vi "rad_Check Firmware.vi"(8 "error in (no error)":errorcluster, 11 "System Configuration":refnum<k21>) -> (0 "error out":errorcluster, 3 "System Configuration out":refnum<k21>, 4 "Bad firmware and user canceled":bool)   [LabVIEW 2016]
uses:
  <resource>/objmgr/nisysapi.rc
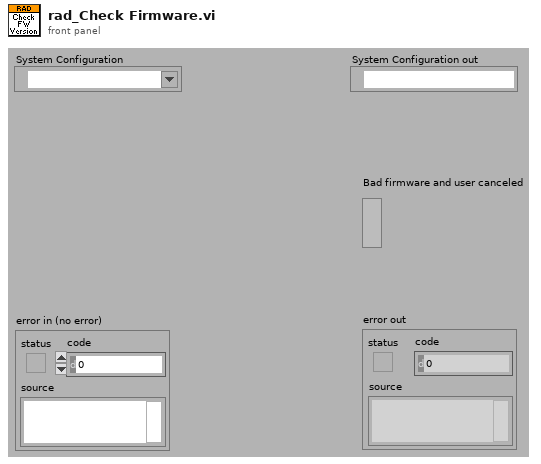
[diagram p1: front panel]
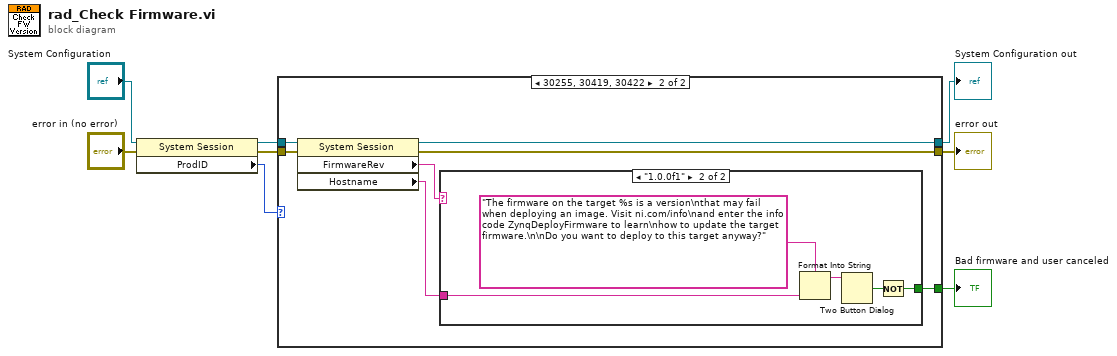
[diagram p0: block diagram]
diagram:
  n1 = property class="System Session"(reference="System Configuration", error in="error in (no error)") -> (reference out=w4:refnum<k21>, error out=w3:errorcluster, "ProdID"=w6:i32)
  n2 = case shown="30255, 30419, 30422" w6 {
    tunnel: [_ w17] -> w5
    tunnel: w4 -> [w10 w16]
    tunnel: w3 -> [w9 w15]
    tunnel: [w10 w14] -> w2
    tunnel: [w9 w13] -> w1
    frame Default {
      # "No other products are known to have problematic\nfirmware versions, as related to deployment."
    }
    frame 30255, 30419, 30422 {
      n3 = property class="System Session"(reference=w16, error in=w15) -> (reference out=w14:refnum<k21>, error out=w13:errorcluster, "FirmwareRev"=w12:string, "Hostname"=w11:string)
      n4 = case shown="\"1.0.0f1\"" w12 {
        tunnel: [_ w21] -> w17
        tunnel: w11 -> [_ w18]
        frame Default {
          # "Assume all other versions of the firmware are fine."
        }
        frame "1.0.0f1" {
          n5 = Format Into String(format string="The firmware on the target %s is a version\nthat may fail when deploying an image. Visit ni.com/info\nand enter the info code ZynqDeployFirmware to learn\nhow to update the target firmware.\n\nDo you want to deploy to this target anyway?", w18) -> (resulting string=w20:string)  [unwired: 2 in, 1 out]
          n6 = Two Button Dialog(message=w20) -> (T button?=w22:bool)  [unwired: 2 in]
          n7 = Not(x=w22) -> (.not. x?=w21:bool)
        }
      }
    }
  }
  "System Configuration out" <- w2
  "error out" <- w1
  "Bad firmware and user canceled" <- w5
